vi "Init(Config) Log CSV File Sink.vi"(7 "CSV File Sink Configuration":T1, 8 "error in (no error)":errorcluster, 9 "iName":string, 10 "iType":string) -> (0 "error out":errorcluster, 3 "CSV File Sink":refnum<class "CSV File Sink.lvclass">)   [LabVIEW 2016, in "Stream Log.lvlib" / "CSV File Sink.lvclass"]
uses:
  <userlib>/Composed Systems/Stream/Log/CSV File Sink/CSV File Sink.lvclass
  C:/Program Files (x86)/National Instruments/LabVIEW 2016/user.lib/Composed Systems/Stream/Actor/Actor Class/Ancestral Actor.lvclass
  C:/Program Files (x86)/National Instruments/LabVIEW 2016/user.lib/Composed Systems/Stream/Log/Text File Sink/Text File Sink.lvclass
  <userlib>/Composed Systems/Stream/Log/Text File Sink/Configuration.ctl
  <userlib>/Composed Systems/Stream/Actor/Actor Class/Ancestral Actor.lvclass/Ancestral Actor.ctl
  <userlib>/Composed Systems/Stream/Log/Text File Sink/Text File Sink.lvclass/Text File Sink.ctl
  <userlib>/Composed Systems/Stream/Actor/Actor Class/Ancestral Actor.lvclass
  <userlib>/Composed Systems/Stream/Log/Text File Sink/Text File Sink.lvclass
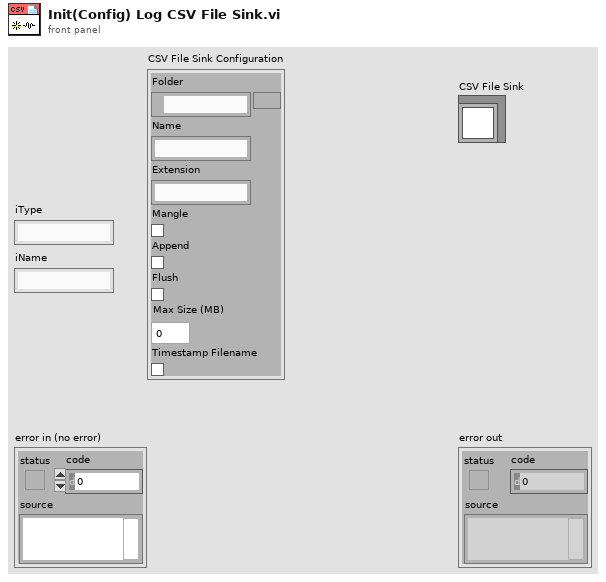
[diagram p1: front panel]
types:
  T1 = typedef "Stream Log.lvlib/Text File Sink.lvclass/Configuration.ctl" = cluster{"Folder":path, "Name":string, "Extension":string, "Mangle":bool, "Append":bool, "Flush":bool, "Max Size (MB)":i64, "Timestamp Filename":bool}
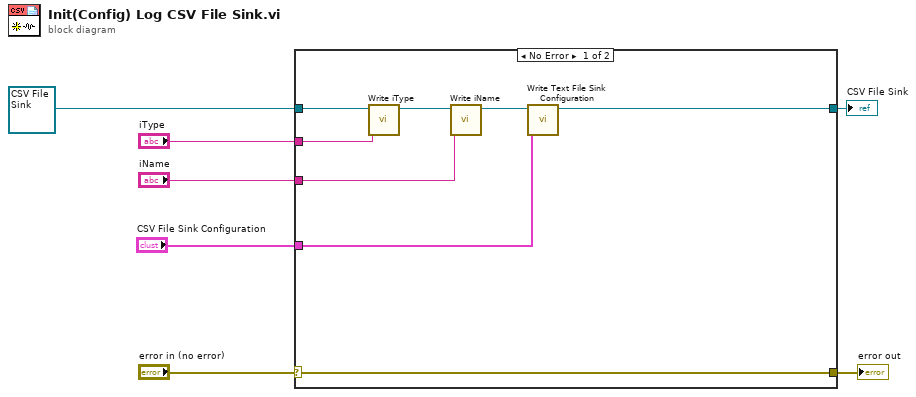
[diagram p0: block diagram]
diagram:
  n1 = case shown="No Error" "error in (no error)" {
    selector: "error in (no error)" -> [w15 w17]
    tunnel: [w15 w17] -> w6
    tunnel: [w9 w16] -> w2
    tunnel: refnum<class "CSV File Sink.lvclass"> refnum ("Stream Log.lvlib:CSV File Sink.lvclass") -> [w14 w16]
    tunnel: "iType" -> [w13 _]
    tunnel: "iName" -> [w11 _]
    tunnel: "CSV File Sink Configuration" -> [w8 _]
    frame No Error {
      n2 = call <userlib>:"Write iType.vi"("iType"=w13, "Ancestral Actor in"=w14) -> ("Ancestral Actor out"=w12:refnum<class "CSV File Sink.lvclass">)  [unwired: 8 in, 1 out]
      n3 = call <userlib>:"Write iName.vi"("iName"=w11, "Ancestral Actor in"=w12) -> ("Ancestral Actor out"=w10:refnum<class "CSV File Sink.lvclass">)  [unwired: 8 in, 1 out]
      n4 = call <userlib>:"Write Text File Sink Configuration.vi"("Text File Sink Configuration"=w8, "Text File Sink in"=w10) -> ("Text File Sink out"=w9:refnum<class "CSV File Sink.lvclass">)  [unwired: 9 in]
    }
    frame Error {
    }
  }
  "error out" <- w6
  "CSV File Sink" <- w2
